vi "AI Read Channel.vi"(1 "Channel":i32, 2 "Device":i32) -> (0 "Value":dbl format="%.3f")   [LabVIEW 2009]
uses:
  <vilib>/Daq/zadvd.llb/AI SingleScan (single-point waveform).vi
panel:
  in  "Case Constant\n(See Context Help)":bool=TRUE
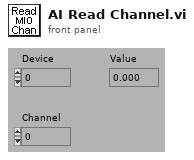
[diagram p1: front panel]
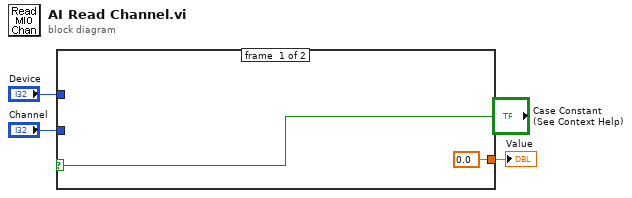
[diagram p0: block diagram]
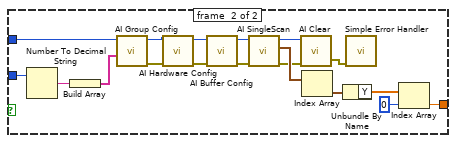
[diagram p2: hidden frame]
diagram:
  n1 = case shown="True" "Case Constant\n(See Context Help)" {
    tunnel: "Device" -> [_ w8]
    tunnel: "Channel" -> [_ w7]
    tunnel: [0.0 w6] -> w2
    frame #0 {
    }
    frame #1 {
      n2 = Number To Decimal String(number=w7) -> (decimal integer string=w9:string)  [unwired: 1 in]
      n3 = Build Array(w9) -> (w10:string[])
      n4 = call <vilib>:"AI Group Config.vi"("channel scan list (empty)"=w10, "device"=w8) -> ("error out"=w17:errorcluster, "task ID"=w20:u32)  [unwired: 7 in, 1 out]
      n5 = call <vilib>:"AI Hardware Config.vi"("error in (no error)"=w17, "task ID"=w20) -> ("error out"=w18:errorcluster, "task ID out"=w21:u32)  [unwired: 7 in, 1 out]
      n6 = call <vilib>:"AI Buffer Config.vi"("error in (no error)"=w18, "task ID"=w21) -> ("error out"=w19:errorcluster, "task ID out"=w22:u32)  [unwired: 8 in]
      n7 = call-poly <vilib>:"AI SingleScan.vi"("error in (no error)"=w19, "task ID"=w22) -> ("error out"=w11:errorcluster, "waveform data"=w13:waveform(dbl)[], "task ID out"=w12:u32)  [unwired: 5 in, 2 out]
      n8 = call <vilib>:"AI Clear.vi"("error in (no error)"=w11, "taskID in"=w12) -> ("error out"=w23:errorcluster)  [unwired: 4 in, 1 out]
      n9 = Index Array(array=w13) -> (element=w14:waveform(dbl))  [unwired: 1 in]
      n10 = Unbundle By Name(w14) -> ("Y"=w15:dbl[])
      n11 = call <vilib>:"Simple Error Handler.vi"("error in (no error)"=w23) -> ()  [unwired: 4 in, 5 out]
      n12 = Index Array(array=w15, index=0 ("Index")) -> (element=w6:dbl)
    }
  }
  "Value" <- w2
